vi "Open.vi"(4 "Notatka refnum":refnum<vi>, 6 "Tytul refnum":refnum<vi>, 9 "Active Row":i32, 10 "Tytuły":string[](array[string]), 11 "Folder":path) -> ()   [LabVIEW 2020]
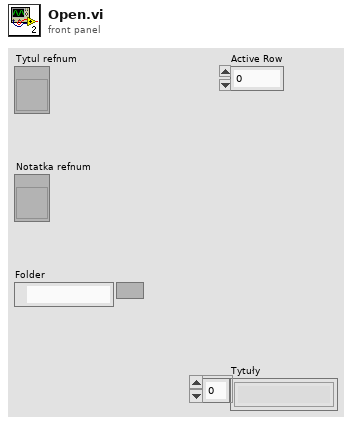
[diagram p1: front panel]
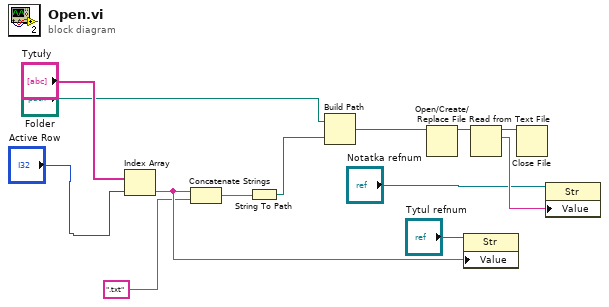
[diagram p0: block diagram]
diagram:
  n1 = Index Array(array="Tytuły", index="Active Row") -> (element=w12:string)
  n2 = Concatenate Strings(w12, ".txt" ("string")) -> (w4:string)
  n3 = String To Path(string=w4) -> (path=w5:path)
  n4 = Build Path(base path="Folder", name or relative path=w5) -> (appended path=w6:path)
  n5 = Open/Create/Replace File(file path (use dialog)=w6) -> (refnum out=w7:refnum<file>)  [unwired: 5 in, 2 out]
  n6 = property on="Property Node" class="Str"(reference="Tytul refnum", "Value"=w12) -> ()  [unwired: 1 in, 2 out]
  n7 = Read from Text File(file (use dialog)=w7) -> (refnum out=w8:refnum<file>, text=w13:string)  [unwired: 3 in, 2 out]
  n8 = Close File(refnum=w8) -> ()  [unwired: 1 in, 2 out]
  n9 = property on="Property Node" class="Str"(reference="Notatka refnum", "Value"=w13) -> ()  [unwired: 1 in, 2 out]
